vi "Dashboard Main.vi"() -> ()   [LabVIEW 2018]
uses:
  CustomThings/Routine.ctl
  CustomThings/StartingLocation.ctl
  CustomThings/Height.ctl
  CustomThings/Piece.ctl
  CustomThings/NumberOfPiecesToScore.ctl
  <vilib>/Rock Robotics/WPI/Camera/WPI_CameraExposure Values.ctl
  <vilib>/Rock Robotics/WPI/Camera/WPI_CameraWhite Balance Values.ctl
  <vilib>/Utility/miscctls.llb/LVRowAndColumnTypeDef.ctl
  <vilib>/event_ctls.llb/eventvkey.ctl
  <vilib>/Rock Robotics/Network Tables/NT Read Numeric Array.vi
  <vilib>/Rock Robotics/WPI/Dashboard/WPI_DashboardLogging Global.vi
  <vilib>/Rock Robotics/Network Tables/NT Write Boolean.vi
  <vilib>/Rock Robotics/Network Tables/NT Read Boolean.vi
panel:
  out "NT Connection":bool
  in  "Camera Settings Right":T1={"Frame Rate"=15, "Compression"=30, "Size"=1, "DB Camera Config"=FALSE} {"Frame Rate" scale=1.0..30.0; "Compression" scale=100.0..-1.0; "Size" items=["640x480", "320x240", "160x120"]}
  in  "Camera Name Right":string(combo)="No Camera Selection"
  out "Camera Perf":string="                          "
  in  "Camera Settings":T1={"Frame Rate"=10, "Compression"=66, "Size"=2, "DB Camera Config"=FALSE} {"Frame Rate" scale=1.0..30.0; "Compression" scale=100.0..-1.0; "Size" items=["640x480", "320x240", "160x120"]}
  in  "TCP":refnum<k5>
  in  "Rec Mode":enum32{"Stop", "Record", "Playback"}(radio)
  out "Robot IP":string
  out "Image Message":string="Timeout in Camera Communications"
  in  "Dashboard Tab":T2(tab)=enum."Custom"
  out "LEDs":u32(colorbox)
  out "ArmHeight":dbl(slide) scale=0.0..100.0
  out "HatchLimitSwitch":bool
  out "LimitSwitchBottom":bool
  out "LimitSwitchTop":bool
  out "Mode":T3(ring)=enum."Disconnected"
  out "Right Camera Perf":cluster{"Bandwidth (Mbps)":dbl, "FPS":dbl}
  in  "Reset":bool
  out "LeftEncoder":dbl
  out "RightEncoder":dbl
  out "Gyro":dbl(knob) scale=-180.0..180.0
  in  "Pieces  to Score":T4=enum."3"
  in  "Rocket Level":T5
  in  "Delay":dbl
  in  "Starting Position":T6
  in  "Routine":T7
  in  "Battery Number":string
  out "Starting Piece":T8=enum."Hatch Panel"
  out "Camera Image Right":T9(plugin-control)
  in  "DB/String 9":string
  in  "DB/String 8":string
  in  "DB/String 7":string
  in  "DB/String 6":string
  in  "DB/String 5":string
  in  "DB/String 4":string
  in  "DB/String 3":string
  in  "DB/String 2":string
  in  "DB/String 1":string
  in  "DB/String 0":string
  in  "DB/Slider 0":dbl(slide) scale=0.0..5.0
  in  "DB/Slider 1":dbl(slide) scale=0.0..5.0
  in  "DB/Slider 2":dbl(slide) scale=0.0..5.0
  in  "DB/Slider 3":dbl(slide) scale=0.0..5.0
  out "DB/LED 3":bool
  out "DB/LED 2":bool
  out "DB/LED 1":bool
  out "DB/LED 0":bool
  in  "DB/Button 3":bool
  in  "DB/Button 2":bool
  in  "DB/Button 1":bool
  in  "DB/Button 0":bool caption="New Name"
  in  "Test Slider":dbl(slide) scale=0.0..100.0 scale format="%#_3g"
  in  "On/Off":bool caption="Solenoid"
  in  "Test Name":u16(ring) items=["Select the test to run..."]
  in  "Test Tree":string(tree)
  in  "Motor":cluster{"Value":dbl, "Enable":bool} {"Value" scale=-1.0..1.0 scale format="%#_3g"}
  out "Progress":T10 {"Test Progress" scale=0.0..100.0}
  in  "Rev/Fwd":cluster{"Forward":bool, "Reverse":bool}
  in  "Test Ring":u16(ring) items=["Monochrome", "Color"]
  out "Cmd Status":string
  in  "Execute Command":bool
  in  "Command Params":string[][](table)
  in  "Command Selection":i32(listbox)
  in  "CheckList":i32(listbox)
  out "Tree":string(tree)
  out "Camera Image":T9(plugin-control)
  in  "Camera Name":string(combo)="No Camera Selection"
  # "HW"
  # "HW"
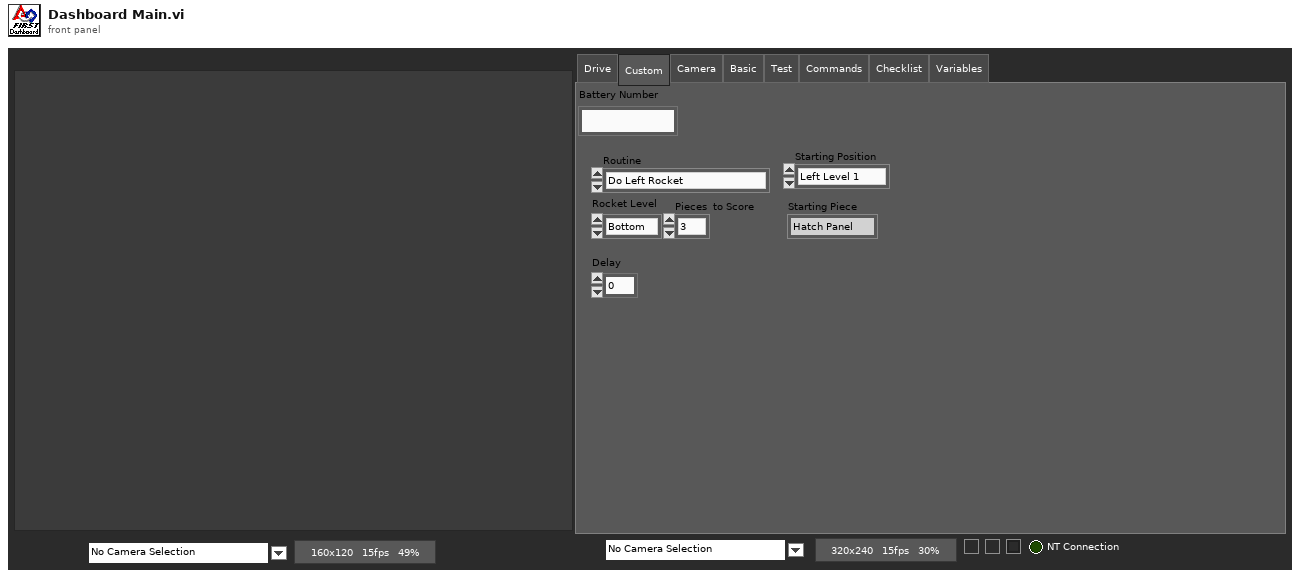
[diagram p1: front panel]
types:
  T1 = cluster{"Frame Rate":i32, "Compression":i32, "Size":u16, "DB Camera Config":bool}
  T2 = enum32{"Drive", "Custom", "Camera", "Basic", "Test", "Commands", "Checklist", "Variables"}
  T3 = enum8{"Tele-Op Disabled", "Tele-Op Enabled", "Auto Disabled", "Auto Enabled", "Test Disabled", "Test Enabled", "Disconnected", "No Code", "E-Stop"}
  T4 = typedef "NumberOfPiecesToScore.ctl" = enum16{"1", "2", "3", "4"}
  T5 = typedef "Height.ctl" = enum16{"Bottom", "Middle", "Top"}
  T6 = typedef "StartingLocation.ctl" = enum16{"Left Level 1", "Center Level 1", "Right Level 1", "Left Level 2", "Right Level 2"}
  T7 = typedef "Routine.ctl" = enum16{"Do Left Rocket", "Do Right Rocket", "Do Left Cargo Ship Panels", "Do Right Cargo Ship Panels", "Do Front Left Cargo Ship", "Do Front Right Cargo Ship", "Do Teleop"}
  T8 = typedef "Piece.ctl" = enum16{"None", "Cargo", "Hatch Panel"}
  T9 = typedef "IMAQ Image.ctl" = refnum<image>
  T10 = cluster{"Test Progress":u8, "Test Progress Text":string}
  T11 = cluster{"Save Path":path, "Interval (s)":dbl, "Keep":i32}
  T12 = typedef "Image Type" = u32
  T13 = cluster{"IDs":cluster{"RPC field ID":u16, "Unique ID":u16}, "String":string}
  T14 = cluster{"Error Strings":string, "Disable Counts":cluster{u16, u16}, "Rail Faults":cluster{u16, u16, u16}, "Robot IP":string, "DB Mode":u8, "Event Info":cluster{"Name":string, "Type":u8, "Number":u16, "Replay":u8}}
  T15 = cluster{"Storage":cluster{"Disk Free":u64, "RAM Block":u32, "RAM free":u32}, "CPU Utilization":cluster{"CPU % ISR":sgl, "CPU % Time Crit":sgl, "CPU % Timed Str":sgl, "CPU % High":sgl, "CPU % Above":sgl, "CPU % Normal":sgl, "CPU % Low":sgl}, "CAN":cluster{"% Bus Utilization":sgl, "Bus Off Cnt":u32, "TX_FIFO Full Cnt":u32, "Receive Error Cnt":u8, "Transmit Error Cnt":u8}, "HID":cluster{"HID Outputs":u32, "Rumble Low":u16, "Rumble High":u16}[]}
  T16 = cluster{"Status bits":cluster{"Test Mode":bool, "Autonomous":bool, "Enabled":bool, "Code Start":bool, "Brownout":bool, "Reserved 2":bool, "Reserved 3":bool, "E-Stop":bool}, "Code Trace":cluster{"Disabled":bool, "TeleOp":bool, "Auto":bool, "Test":bool}, "Controller Type":enum16{"unknown", "cRIO", "roboRio"}, "Code?":enum16{"unknown", "noCode", "code"}, "Battery V":dbl}
  T17 = cluster{"Control Bits":cluster{"TestMode":bool, "Autonomous":bool, "Enabled":bool, "FMS Present":bool, bool, bool, bool, "E-Stop":bool}, "Team Station ":u8, "Countdown":sgl, "Joystick Values":cluster{"Axes":dbl[], "Buttons":bool[], "POVs":i16[]}[]}
  T18 = cluster{"Axes":dbl[], "Buttons":bool[], "POVs":i16[]}[]
  T19 = cluster{"Axes":dbl[], "Buttons":bool[], "POVs":i16[]}
  T20 = cluster{"Camera Image":refnum<vi>, "Dashboard Tab":refnum<vi>, "Rec Mode":refnum<vi>, "Test Slider":refnum<vi>, "On/Off ":refnum<vi>, "Test Ring":refnum<vi>, "Rev/Fwd":refnum<vi>, "Test Name":refnum<vi>, "Motor":refnum<vi>, "Progress":refnum<vi>, "CheckList":refnum<vi>, "Tree":refnum<vi>, "Test Tree":refnum<vi>, "Command Params":refnum<vi>, "Command Selection":refnum<vi>, "Execute Command":refnum<vi>, "Cmd Status":refnum<vi>, "Camera Settings":refnum<vi>, "Camera Name":refnum<vi>, "Camera Perf":refnum<vi>, "Camera Settings Right":refnum<vi>, "Camera Name Right":refnum<vi>, "Camera Image Right":refnum<vi>}
  T21 = typedef "WPI_CameraExposure Values.ctl" = enum16{"Auto", "Flicker-free 50 Hz", "Flicker-free 60 Hz", "Hold current", "Custom"}
  T22 = typedef "WPI_CameraWhite Balance Values.ctl" = enum16{"Auto", "Fixed indoor", "Fixed outdoor 1", "Fixed outdoor 2", "Fixed fluorescent 1", "Fixed fluorescent 2", "Hold current", "Custom"}
  T23 = cluster{"Exposure":T21, "Exposure (%)":dbl, "Brightness":i32, "White Balance":T22, "Color Temp (K)":dbl}
  T24 = cluster{"Global Rectangle":i32[], "Contours":cluster{"Contour Type":u32, "ROI Type":u32, "Points":i32[]}[]}
  T25 = cluster{"Camera Name":string, string, "Saved DB Images Info":cluster{"Save Path":path, "Interval (s)":dbl, "Keep":i32}}
  T26 = cluster{"Camera Name Right":string, string, "Saved DB Images Info":cluster{"Save Path":path, "Interval (s)":dbl, "Keep":i32}}
  T27 = cluster{"Operation":enum16{"Update", "Clear"}, "Color Box":u32}[]
  T28 = typedef "eventvkey.ctl" = enum16{"ASCII", "Enter", "Return", "Shift", "Ctrl", "Alt", "Cmd", "Opt", "Caps", "NumLock", "Clear", "Break", "Up", "Down", "Left", "Right", "Insert", "Delete", "Home", "End", "PageUp", "PageDown", "Escape", "Help", "Pause", "ScrollLock", "F1", "F2", "F3", "F4", "F5", "F6", "F7", "F8", "F9", "F10", "F11", "F12", "F13", "F14", "F15", "F16", "F17", "F18", "F19", "F20", "F21", "F22", "F23", "F24", "Play", "VolumeUp", "VolumeDown", "Mute", "Two Byte Char"}
  T29 = cluster{"Image Size":bool, "Image Type":bool, "Pixel Value":bool, "ROI Information":bool, "Zoom Factor":bool}
  T30 = cluster{"Operation":enum16{"Update", "Clear"}, "Color Box":u32}
  T31 = typedef "LVRowAndColumnTypeDef.ctl" = cluster{"Row":i32, "Column":i32}
  T32 = cluster{"Shift":bool, "Ctrl":bool, "Alt":bool, "Cmd":bool, "Opt":bool}
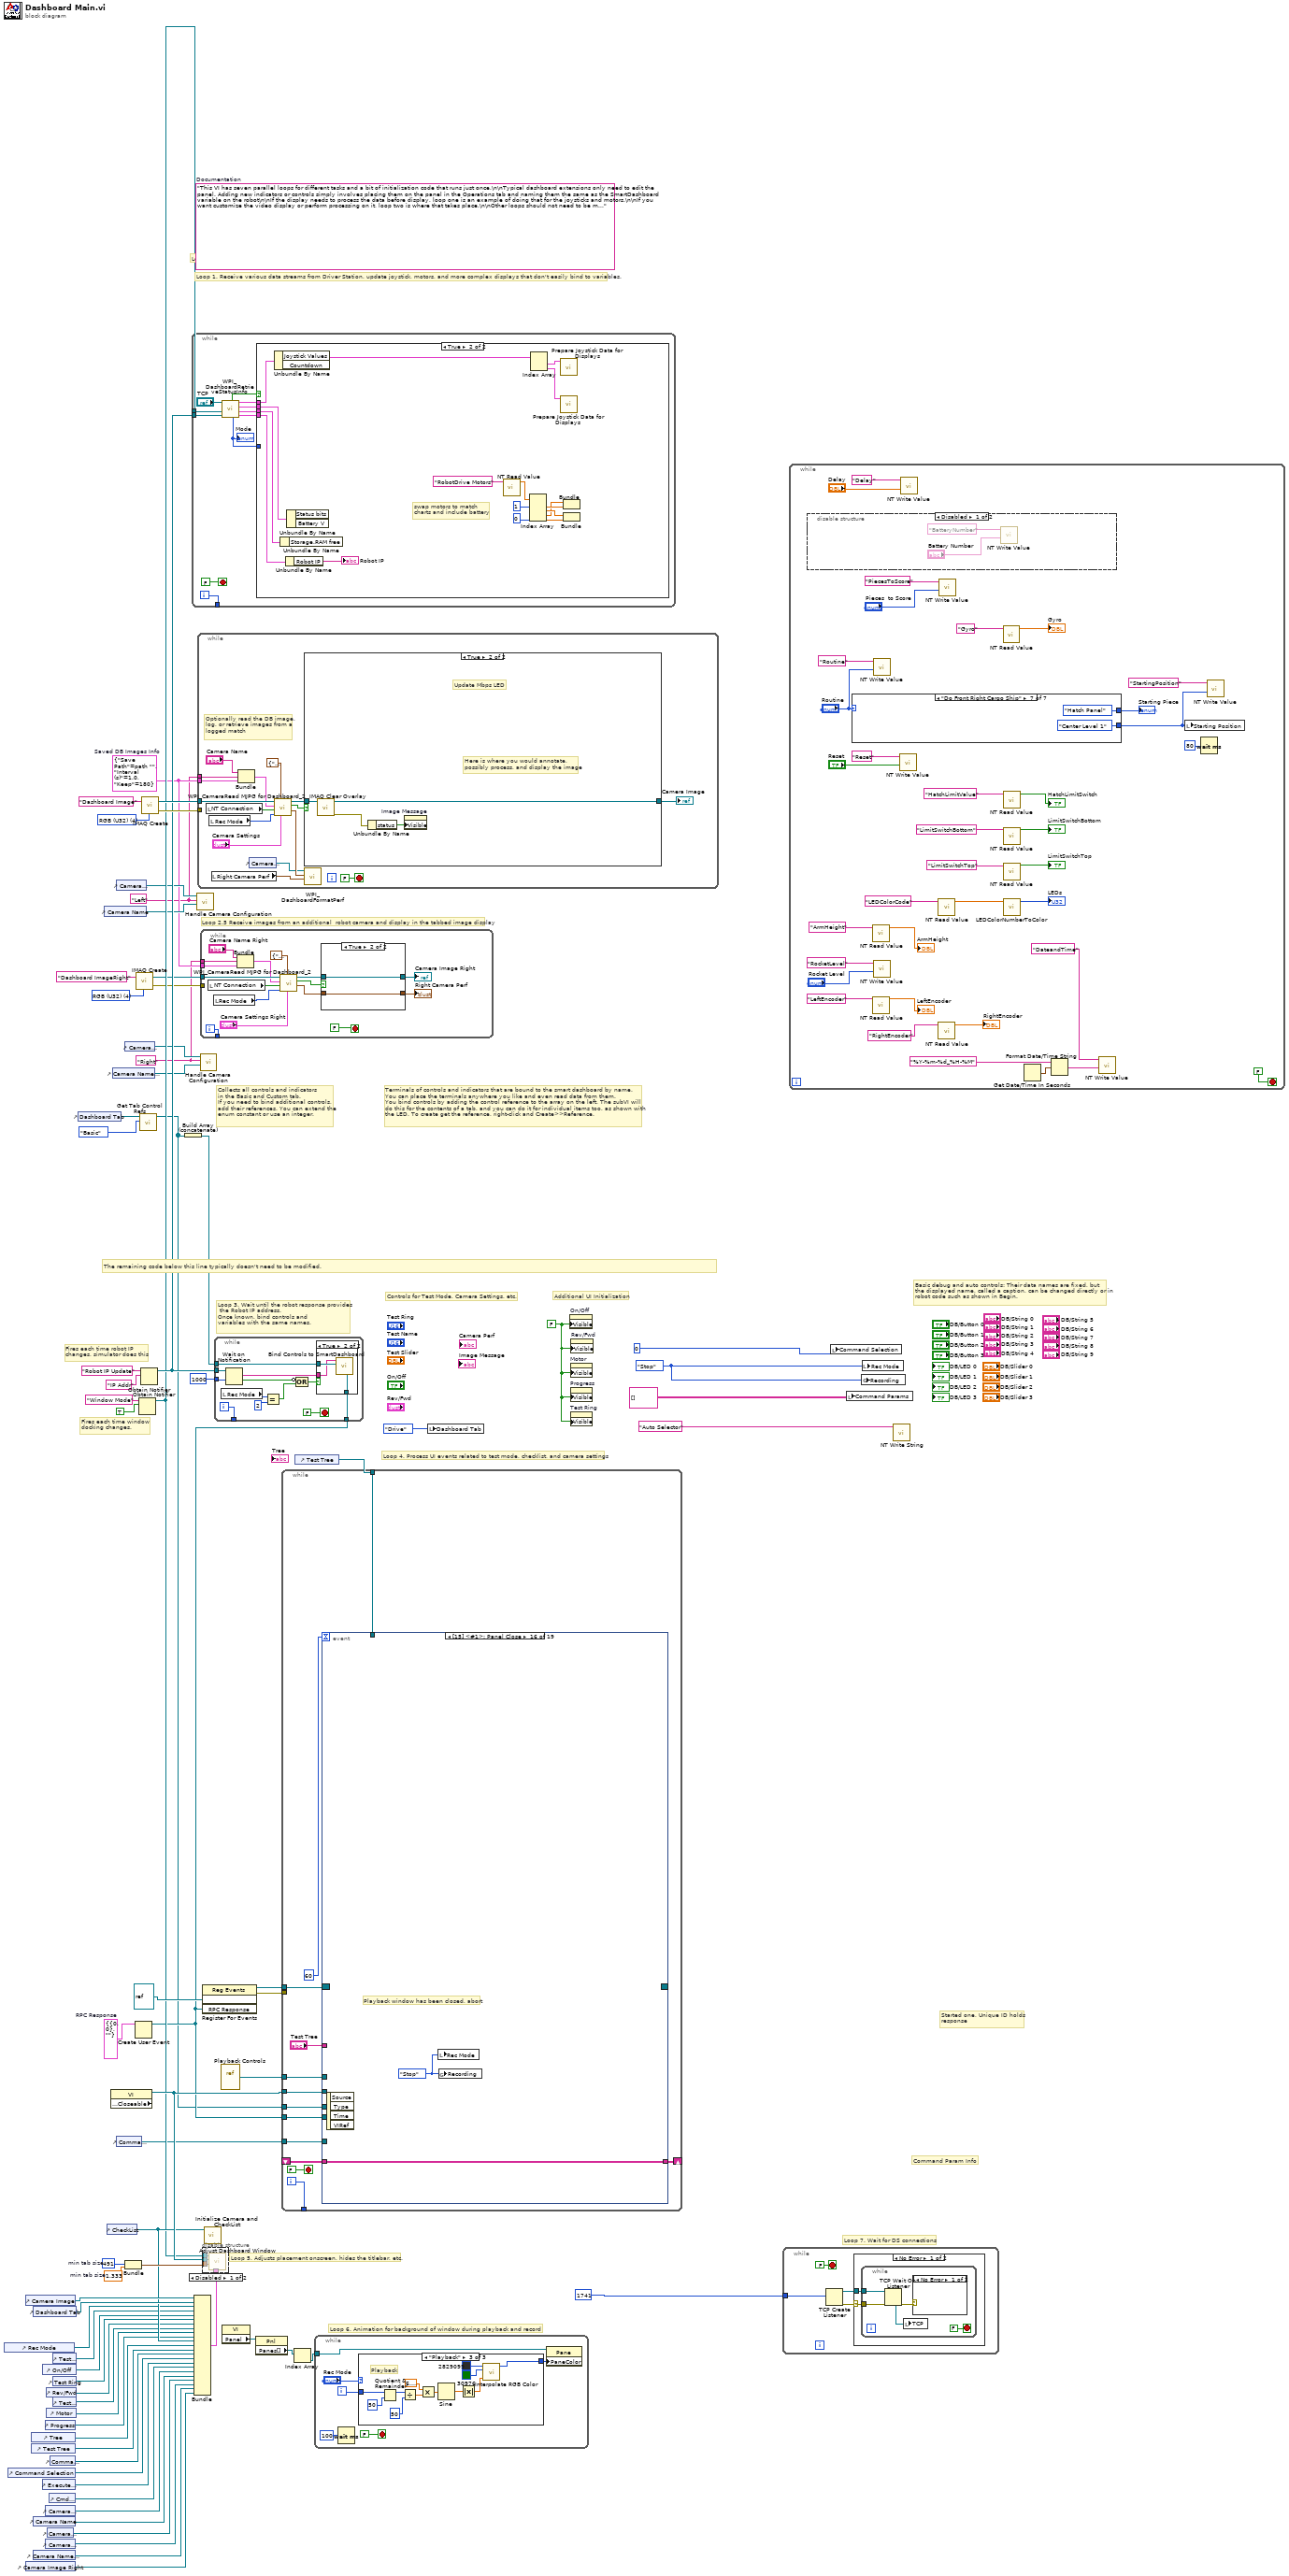
[diagram p0: block diagram]
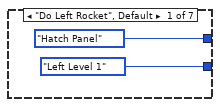
[diagram p2: hidden frame]
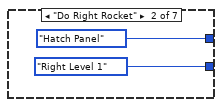
[diagram p3: hidden frame]
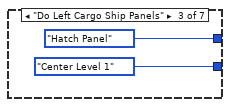
[diagram p4: hidden frame]
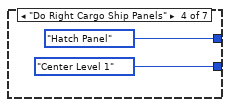
[diagram p5: hidden frame]
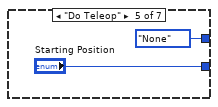
[diagram p6: hidden frame]
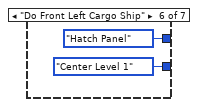
[diagram p7: hidden frame]
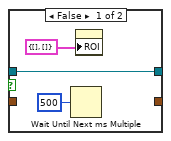
[diagram p10: hidden frame]
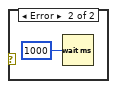
[diagram p11: hidden frame]
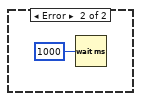
[diagram p12: hidden frame]
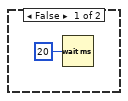
[diagram p13: hidden frame]
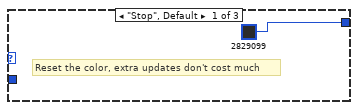
[diagram p14: hidden frame]
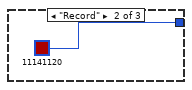
[diagram p15: hidden frame]
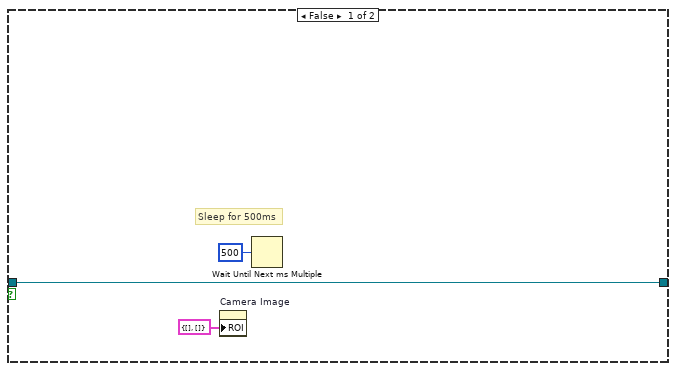
[diagram p17: hidden frame]
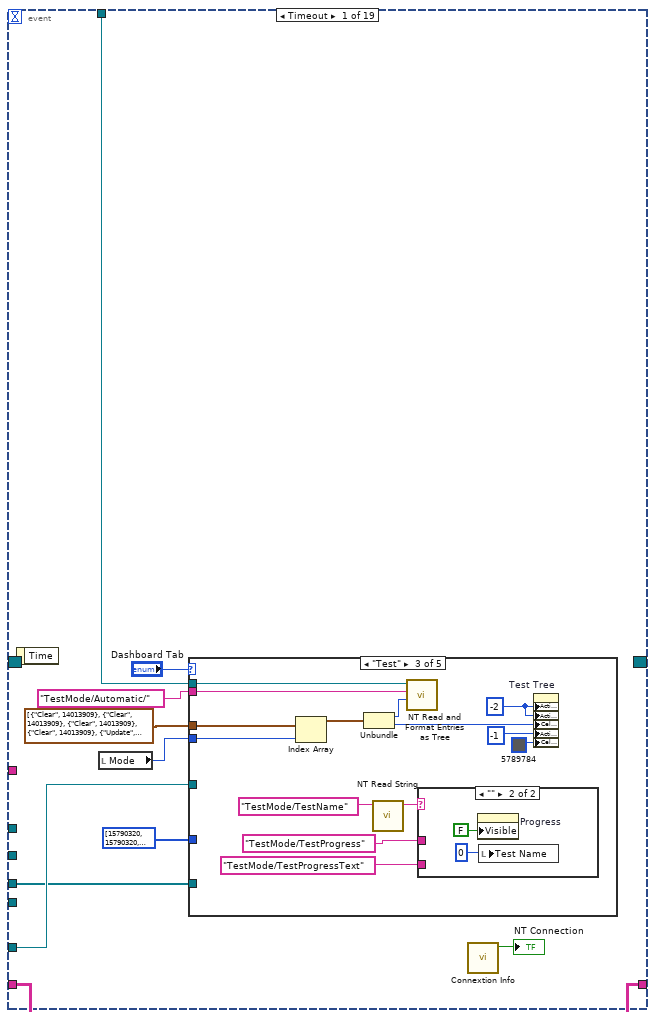
[diagram p18: hidden frame]
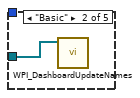
[diagram p20: hidden frame]
diagram:
  w4 = T11 {"Save Path"=path "", "Interval (s)"=1.0, "Keep"=180}  # Saved DB Images Info
  w3 = "Right"
  w2 = "Left"
  w12 = T12 4 items=["Grayscale (U8)", "Grayscale (I16)", "Grayscale (SGL)", "Complex (CSG)", "RGB (U32)", "HSL (U32)", "RGB (U64)"] ("Image Type")
  w27 = T13 {"IDs"={"RPC field ID"=0, "Unique ID"=0}, "String"=""}  # RPC Response
  w49 = 491  # min tab size
  w48 = 1.333  # min tab size
  w55 = enum32{"Stop", "Record", "Playback"}."Stop" ("Rec Mode")
  w34 = FALSE ("Visible")
  (unwired) "This VI has seven parallel loops for different tasks and a bit of initialization code that runs just once.\n\nTypical dashboard extensions only need to edit the panel. Adding new indicators or controls simply involves placing them on the panel in the Operations tab and naming them the same as the SmartDashboard variable on the robot\n\nIf the display needs to process the data before display, loop one is an example of doing that for the joysticks and motors.\n\nIf you want customize the video display or perform processing on it, loop two is where that takes place.\n\nOther loops should not need to be modified. They are pretty standard, and document the task they perform."  # Documentation
  w72 = T12 4 items=["Grayscale (U8)", "Grayscale (I16)", "Grayscale (SGL)", "Complex (CSG)", "RGB (U32)", "HSL (U32)", "RGB (U64)"] ("Image Type")
  # "Loop 2.5 Receive images from an additional  robot camera and display in the tabbed image display"
  # "Command Param Info"
  # "Started one, Unique ID holds\nresponse"
  # "Loop 7. Wait for DS connections"
  # "Basic debug and auto controls: Their data names are fixed, but\nthe displayed name, called a caption, can be changed directly or in\nrobot code such as shown in Begin."
  # "Controls for Test Mode, Camera Settings, etc."
  # "Additional UI Initialization"
  # "Loop 6. Animation for background of window during playback and record"
  # "Fires each time robot IP\nchanges, simulator does this"
  # "Fires each time window\ndocking changes."
  # "Collects all controls and indicators\nin the Basic and Custom tab.\nIf you need to bind additional controls,\nadd their references. You can extend the\nenum constant or use an integer."
  # "The remaining code below this line typically doesn't need to be modified."
  # "Loop 4. Process UI events related to test mode, checklist, and camera settings"
  # "Terminals of controls and indicators that are bound to the smart dashboard by name.\nYou can place the terminals anywhere you like and even read data from them.\nYou bind controls by adding the control reference to the array on the left. The subVI will\ndo this for the contents of a tab, and you can do it for individual items too, as shown with\nthe LED. To create get the reference, right-click and Create>>Reference."
  # "Loop 3. Wait until the robot response provides\n the Robot IP address.\nOnce known, bind controls and\nvariables with the same names."
  # "Loop 5. Adjusts placement onscreen, hides the titlebar, etc."
  # "Loop 1. Receive various data streams from Driver Station, update joystick, motors, and more complex displays that don't easily bind to variables."
  # "Loop 2. Receive primary camera images from robot, update Mbps, fps, and do any processing or display"
  n1 = control-ref of="Rec Mode"() -> (w40:refnum<vi>)
  n2 = control-ref of="Command Selection"() -> (w26:refnum<vi>)
  n3 = control-ref of="Camera Image Right"() -> (w5:refnum<vi>)
  n4 = control-ref of="Camera Image"() -> (w51:refnum<vi>)
  n5 = control-ref of="Tree"() -> (w44:refnum<vi>)
  n6 = control-ref of="Test Tree"() -> (w43:refnum<vi>)
  n7 = control-ref of="Dashboard Tab"() -> (w50:refnum<vi>)
  n8 = control-ref of="Camera Name"() -> (w17:refnum<vi>)
  n9 = control-ref of="Camera Name Right"() -> (w6:refnum<vi>)
  n10 = control-ref of="Execute Command"() -> (w28:refnum<vi>)
  n11 = control-ref of="On/Off"() -> (w38:refnum<vi>)
  n12 = control-ref of="Progress"() -> (w35:refnum<vi>)
  n13 = control-ref of="Camera Settings"() -> (w18:refnum<vi>)
  n14 = control-ref of="Camera Settings Right"() -> (w7:refnum<vi>)
  n15 = control-ref of="Rev/Fwd"() -> (w36:refnum<vi>)
  n16 = control-ref of="Motor"() -> (w41:refnum<vi>)
  n17 = control-ref of="Camera Perf"() -> (w16:refnum<vi>)
  n18 = control-ref of="Cmd Status"() -> (w22:refnum<vi>)
  n19 = control-ref of="Command Params"() -> (w29:refnum<vi>)
  n20 = control-ref of="Test Slider"() -> (w39:refnum<vi>)
  n21 = control-ref of="Test Ring"() -> (w37:refnum<vi>)
  n22 = control-ref of="Test Name"() -> (w42:refnum<vi>)
  n23 = control-ref of="Dashboard Tab"() -> (w53:refnum<vi>)
  n24 = control-ref of="Camera Name"() -> (w19:refnum<vi>)
  n25 = control-ref of="CheckList"() -> (w45:refnum<vi>)
  n26 = property class="VI" props=["Front Panel.Closeable"]() -> (reference out=w54:refnum<vi>)  [unwired: 2 in, 2 out]
  n27 = control-ref of="Camera Name Right"() -> (w8:refnum<vi>)
  n28 = control-ref of="Camera Settings"() -> (w20:refnum<vi>)
  n29 = control-ref of="Command Params"() -> (w21:refnum<vi>)
  n30 = control-ref of="Camera Settings Right"() -> (w9:refnum<vi>)
  n31 = Bundle("min tab size"=w49, "min tab size"=w48) -> (w47:cluster{"min tab size":i32, "min tab size":dbl})  [unwired: 1 in]
  n32 = Create User Event(user event datatype=w27) -> (user event=w23:refnum<user-event>)  [unwired: 1 in, 1 out]
  n33 = call "IMAQ Create"("Image Name"="Dashboard ImageRight", "Image Type"=w12) -> ("New Image"=w11:T9, "error out"=w10:errorcluster)  [unwired: 2 in, 1 out]
  n34 = Obtain Notifier(name (unnamed)="Window Mode", notification data type=TRUE) -> (notifier out=w32:refnum<notifier>)  [unwired: 2 in, 2 out]
  n35 = call <vilib>:"Get Tab Control Refs.vi"("Page Index"=T2."Basic" ("Dashboard Tab"), "TabControl in"=w53) -> ("ControlsOnPage"=w15:refnum<vi>[])  [unwired: 9 in]
  n36 = Obtain Notifier(name (unnamed)="Robot IP Update", notification data type="IP Addr" ("name (unnamed)")) -> (notifier out=w33:refnum<notifier>)  [unwired: 2 in, 2 out]
  n37 = call "IMAQ Create"("Image Name"="Dashboard Image", "Image Type"=w72) -> ("New Image"=w70:T9, "error out"=w69:errorcluster)  [unwired: 2 in, 1 out]
  n38 = Build Array (concatenate)(w15) -> (w52:refnum<vi>[])
  n39 = while {
    tunnel: [w82] -> _
    tunnel: w33 -> [w76]
    tunnel: w32 -> [w73]
    i -> [w82]
    stop <- FALSE stop-if-true
    n40 = call <vilib>:"WPI_DashboardRetrieveStatusInfo.vi"("Binding Refnum"=w76, "Window Mode Notifier"=w73, "TCP Cnx"="TCP") -> ("Power and Errors"=w77:T14, "Robot Metrics"=w80:T15, "Status Info"=w81:T16, "Control Info"=w78:T17, "Robot Mode"=w75:T3, "Process?"=w79:bool)  [unwired: 3 in]
    "Mode" <- w75
    n41 = case shown="True" w79 {
      tunnel: w81 -> [_ w100]
      tunnel: w80 -> [_ w99]
      tunnel: w78 -> [_ w98]
      tunnel: w77 -> [_ w97]
      tunnel: w75 -> [_ _]
      frame False {
        n42 = Wait (ms)(milliseconds to wait=u32 20) -> ()  [unwired: 1 out]
      }
      frame True {
        # "swap motors to match\ncharts and include battery"
        n43 = Unbundle By Name(w98) -> ("Joystick Values"=w90:T18)  [unwired: 1 out]
        n44 = Unbundle By Name(w99) -> ()  [unwired: 1 out]
        n45 = Unbundle By Name(w97) -> ("Robot IP"=→"Robot IP":string)
        n46 = Unbundle By Name(w100) -> ()  [unwired: 2 out]
        n47 = call-poly <vilib>:"NT Read Value.vi"("Name"="RobotDrive Motors") -> ("Numeric Array"=w86:dbl[])  [unwired: 9 in, 1 out]
        n48 = Index Array(array=w86, index #1=1, index #4=0) -> (element #1=w92:dbl, element #2=w93:dbl, element #3=w91:dbl, element #4=w96:dbl)  [unwired: 2 in]
        n49 = Index Array(array=w90) -> (element #1=w89:T19, element #2=w88:T19)  [unwired: 2 in]
        n50 = call "Prepare Joystick Data for Displays.vi"("Joystick Values"=w88) -> ()  [unwired: 8 in, 3 out]
        n51 = call "Prepare Joystick Data for Displays.vi"("Joystick Values"=w89) -> ()  [unwired: 8 in, 3 out]
        n52 = Bundle("Numeric"=w91, "Numeric"=w92) -> ()  [unwired: 1 in, 1 out]
        n53 = Bundle("Numeric"=w93, "Numeric"=w96) -> ()  [unwired: 1 in, 1 out]
      }
    }
  }
  n54 = Bundle("Camera Image"=w51, "Dashboard Tab"=w50, "Rec Mode"=w40, "Test Slider"=w39, "On/Off"=w38, "Test Ring"=w37, "Rev/Fwd"=w36, "Test Name"=w42, "Motor"=w41, "Progress"=w35, "CheckList"=w45, "Tree"=w44, "Test Tree"=w43, "Command Params"=w29, "Command Selection"=w26, "Execute Command"=w28, "Cmd Status"=w22, "Camera Settings"=w18, "Camera Name"=w17, "Camera Perf"=w16, "Camera Settings Right"=w7, "Camera Name Right"=w6, "Camera Image Right"=w5) -> (w46:T20)  [unwired: 1 in]
  n55 = call "Handle Camera Configuration.vi"("CameraNameRef"=w19, "Display Name"=w2, "ClusterRef"=w20) -> ()  [unwired: 9 in]
  n56 = while {
    tunnel: w70 -> [w115]
    tunnel: w69 -> [_]
    tunnel: w4 -> [w108]
    tunnel: w2 -> [w105]
    stop <- FALSE stop-if-true
    # "Optionally read the DB image,\nlog, or retrieve images from a\nlogged match"
    n57 = local read "NT Connection"() -> (w109:bool)
    n58 = local read "Rec Mode"() -> (w112:enum32{"Stop", "Record", "Playback"})
    n59 = local read "Right Camera Perf"() -> (w103:cluster{"Bandwidth (Mbps)":dbl, "FPS":dbl})
    n60 = Bundle("Camera Name"="Camera Name", w105, "Saved DB Images Info"=w108) -> (w107:T25)  [unwired: 1 in]
    n61 = control-ref of="Camera Perf"() -> (w102:refnum<vi>)
    n62 = call <vilib>:"WPI_CameraRead MJPG for Dashboard_2.vi"("Camera Settings"="Camera Settings", "Camera Settings 2"=T23 {"Exposure"=enum."Custom", "Exposure (%)"=75.0, "Brightness"=50, "White Balance"=enum."Custom", "Color Temp (K)"=0.0}, "Rec Mode"=w112, "NT Connection"=w109, "Capture Info"=w107, "Image in"=w115) -> ("perf info"=w104:cluster{"Bandwidth (Mbps)":dbl, "fps":dbl}, "Active"=w113:bool, "Image\\ out"=w114:T9)  [unwired: 3 in]
    n63 = case shown="True" w113 {
      tunnel: w114 -> [w118 w121]
      tunnel: [w118 w120] -> w110
      frame False {
        # "Sleep for 500ms"
        n64 = property on="Camera Image" class="ImageControl"("ROI"=T24 {"Global Rectangle"=[], "Contours"=[]}) -> ()  [unwired: 2 in, 2 out]
        n65 = Wait Until Next ms Multiple(millisecond multiple=u32 500) -> ()  [unwired: 1 out]
      }
      frame True {
        # "Here is where you would annotate,\npossibly process, and display the image"
        # "Update Mbps LED"
        n66 = call "IMAQ Clear Overlay"("Image"=w121) -> ("error out"=w122:errorcluster, "Image Out"=w120:T9)  [unwired: 2 in, 7 out]
        n67 = Unbundle By Name(w122) -> ("status"=w123:bool)
        n68 = property on="Image Message" class="Str"("Visible"=w123) -> ()  [unwired: 2 in, 2 out]
      }
    }
    "Camera Image" <- w110
    n69 = call <vilib>:"WPI_DashboardFormatPerf.vi"("Right Camera Perf"=w103, "Performance"=w104, "String in"=w102) -> ()  [unwired: 9 in]
  }
  n70 = while {
    tunnel: w11 -> [w139]
    tunnel: w10 -> [_]
    tunnel: [w134] -> _
    tunnel: w4 -> [w130]
    tunnel: w3 -> [w127]
    i -> [w134]
    stop <- FALSE stop-if-true
    n71 = local read "NT Connection"() -> (w131:bool)
    n72 = local read "Rec Mode"() -> (w138:enum32{"Stop", "Record", "Playback"})
    n73 = Bundle("Camera Name Right"="Camera Name Right", w127, "Saved DB Images Info"=w130) -> (w129:T26)  [unwired: 1 in]
    n74 = call <vilib>:"WPI_CameraRead MJPG for Dashboard_2.vi"("Camera Settings"="Camera Settings Right", "Camera Settings 2"=T23 {"Exposure"=enum."Custom", "Exposure (%)"=75.0, "Brightness"=50, "White Balance"=enum."Custom", "Color Temp (K)"=0.0}, "Rec Mode"=w138, "NT Connection"=w131, "Capture Info"=w129, "Image in"=w139) -> ("perf info"=w125:cluster{"Bandwidth (Mbps)":dbl, "fps":dbl}, "Active"=w133:bool, "Image\\ out"=w136:T9)  [unwired: 3 in]
    n75 = case shown="True" w133 {
      tunnel: w136 -> [w141 w144]
      tunnel: [w141 w144] -> w132
      tunnel: [_ w143] -> w126
      tunnel: w125 -> [_ w143]
      frame False {
        n76 = Wait Until Next ms Multiple(millisecond multiple=u32 500) -> ()  [unwired: 1 out]
        n77 = property on="Camera Image Right" class="ImageControl"("ROI"=T24 {"Global Rectangle"=[], "Contours"=[]}) -> ()  [unwired: 2 in, 2 out]
      }
      frame True {
      }
    }
    "Camera Image Right" <- w132
    "Right Camera Perf" <- w126
  }
  n78 = call "Handle Camera Configuration.vi"("CameraNameRef"=w8, "Display Name"=w3, "ClusterRef"=w9) -> ()  [unwired: 9 in]
  n79 = register-events(refnum<vi> refnum, w23) -> (reference out=w59:refnum<event-registration>, error out=w58:errorcluster)  [unwired: 2 in]
  n80 = disable-structure shown="Disabled" {
    disable-tunnel: w54 -> [w148 _]
    disable-tunnel: w47 -> [w147 _]
    disable-tunnel: w46 -> [w146 _]
    disable-tunnel: w32 -> [w145 _]
    frame Disabled {
      n81 = call "Adjust Dashboard Window.vi"("Sizing Refnums"=w146, "Size Constraints"=w147, "VI"=w148, "WIn Mode"=w145) -> ()  [unwired: 8 in]
    }
    frame Enabled {
    }
  }
  n82 = call "Initialize Camera and CheckList.vi"("ListBox in"=w45) -> ()  [unwired: 11 in]
  n83 = while {
    tunnel: w52 -> [w160]
    tunnel: w33 -> [w158]
    tunnel: [w156] -> _
    tunnel: u32 1000 ("milliseconds to wait") -> [w155]
    tunnel: w23 -> [w149]
    i -> [w156]
    stop <- FALSE stop-if-true
    n84 = local read "Rec Mode"() -> (w151:enum32{"Stop", "Record", "Playback"})
    n85 = Wait on Notification(notifier=w158, timeout in ms (-1)=w155) -> (notification=w157:string, timed out?=w153:bool)  [unwired: 2 in, 2 out]
    n86 = Equal?(x=w151, y=u16 2 ("Rec Mode")) -> (x = y?=w152:bool)
    n87 = Compound Arithmetic op=OR(invert w153, w152) -> (w154:bool)
    n88 = case shown="True" w154 {
      tunnel: w160 -> [_ w163]
      tunnel: w157 -> [_ w162]
      tunnel: w149 -> [_ w161]
      frame False {
      }
      frame True {
        n89 = call <vilib>:"Bind Controls to SmartDashboard.vi"("RPC ref"=w161, "Bound Control Refs"=w163, "Server IP Address"=w162) -> ()  [unwired: 9 in]
      }
    }
  }
  n90 = vi-ref "Playback Controls.vi"() -> (w60:refnum<vi>)
  n91 = property class="VI"() -> ("Panel"=w62:refnum<vi>)  [unwired: 2 in, 2 out]
  n92 = property class="Pnl"(reference=w62) -> ("Panes[]"=w63:refnum<vi>[])  [unwired: 1 in, 2 out]
  n93 = Index Array(array=w63) -> (element=w61:refnum<vi>)  [unwired: 1 in]
  n94 = control-ref of="Test Tree"() -> (w64:refnum<vi>)
  n95 = while {
    tunnel: [w173] -> _
    tunnel: w64 -> [w172]
    tunnel: w60 -> [w171]
    tunnel: w59 -> [w170]
    tunnel: w58 -> [_]
    tunnel: w54 -> [w169]
    tunnel: w23 -> [w168]
    tunnel: w21 -> [w167]
    shift-right: [w166] -> _
    shift-left: _ -> [w165]
    tunnel: w15 -> [w164]
    i -> [w173]
    stop <- FALSE stop-if-true
    n96 = event shown="[15] <#1>: Panel Close" {
      selector: w170 -> [_ _ _ _ _ _ _ _ _ _ _ _ _ _ _ _ _ _ _]
      dyn-events: [_ _ _ _ _ _ _ _ _ _ _ _ _ _ w427 _ _ _ _] -> _
      timeout: u32 60 ("milliseconds to wait") -> [_ _ _ _ _ _ _ _ _ _ _ _ _ _ _ _ _ _ _]
      tunnel: w172 -> [w185 _ _ _ _ _ _ _ _ _ _ _ _ _ _ _ _ _ _]
      tunnel: "Test Tree" -> [_ _ _ _ _ _ _ _ _ w394 w402 w404 w408 w416 _ _ _ _ _]
      tunnel: w171 -> [_ _ _ _ _ _ _ _ _ _ _ _ _ _ w429 _ w447 _ _]
      tunnel: w169 -> [_ _ _ _ _ _ _ _ _ _ _ _ _ _ w425 _ _ _ _]
      tunnel: w168 -> [_ _ _ _ _ _ _ _ _ _ _ _ _ _ w423 _ _ _ _]
      tunnel: w167 -> [w180 _ _ _ w345 _ _ _ _ _ _ _ _ _ _ _ _ _ _]
      tunnel: [w179 w228 w330 w335 w343 w352 w362 w369 w381 w393 w400 w403 w407 w415 w422 w442 w444 w448 w461] -> w166
      tunnel: w165 -> [w179 w228 w330 w335 w343 _ _ w369 w381 w393 w400 w403 w407 w415 w422 w442 w444 w448 w461]
      tunnel: w164 -> [w177 _ _ _ _ _ _ _ _ _ _ _ _ _ _ _ _ _ _]
      event Timeout {
        n97 = event-data() -> ()  [unwired: 1 in, 1 out]
        n98 = local read "Mode"() -> (w182:T3)
        n99 = case shown="\"Test\"" "Dashboard Tab" {
          tunnel: w185 -> [_ _ w201 _ _]
          tunnel: "TestMode/Automatic/" ("Name Pattern") -> [_ _ w200 _ _]
          tunnel: T27 [{"Operation"=enum."Clear", "Color Box"=14013909}, {"Operation"=enum."Clear", "Color Box"=14013909}, {"Operation"=enum."Clear", "Color Box"=14013909}, {"Operation"=enum."Clear", "Color Box"=14013909}, {"Operation"=enum."Update", "Color Box"=14013909}, {"Operation"=enum."Update", "Color Box"=16777215}, {"Operation"=enum."Clear", "Color Box"=14013909}, {"Operation"=enum."Clear", "Color Box"=14013909}, {"Operation"=enum."Clear", "Color Box"=14013909}] -> [_ _ w193 _ w221]
          tunnel: w182 -> [_ _ w192 _ w220]
          tunnel: u32[] [15790320, 15790320, 15790320, 15790320, 16777215, 16777215, 15790320, 15790320, 15790320] -> [_ _ _ _ w226]
          tunnel: w180 -> [_ _ _ _ w214]
          tunnel: w177 -> [_ w187 _ _ _]
          frame "Custom", Default {
          }
          frame "Basic" {
            n100 = call <vilib>:"WPI_DashboardUpdateNames.vi"("Controls on Tab"=w187) -> ()  [unwired: 11 in]
          }
          frame "Test" {
            w199 = -2 ("Active Item:Row Number")
            n101 = Index Array(array=w193, index=w192) -> (element=w194:T30)
            n102 = Unbundle(w194) -> ("Operation"=w195:enum16{"Update", "Clear"}, "Color Box"=w196:u32)
            n103 = call <vilib>:"NT Read String.vi"("Name"="TestMode/TestName") -> ("String"=w190:string)  [unwired: 9 in, 1 out]
            n104 = call <vilib>:"NT Read and Format Entries as Tree.vi"("Operation"=w195, "Name Pattern"=w200, "Tree Refnum"=w201) -> ()  [unwired: 7 in, 2 out]
            n105 = case shown="\"\"" w190 {
              tunnel: "TestMode/TestProgress" ("Name") -> [w203 _]
              tunnel: "TestMode/TestProgressText" ("Name") -> [w202 _]
              frame Default {
                n106 = call <vilib>:"NT Read Number.vi"("Name"=w203) -> ("Numeric"=w204:dbl)  [unwired: 9 in, 1 out]
                n107 = call <vilib>:"NT Read String.vi"("Name"=w202) -> ("String"=w205:string)  [unwired: 9 in, 1 out]
                n108 = Bundle("Numeric"=w204, "String"=w205) -> (→"Progress":cluster{"Numeric":dbl, "String":string})  [unwired: 1 in]
              }
              frame "" {
                n109 = property on="Progress" class="Clust (strict)"("Visible"=FALSE) -> ()  [unwired: 2 in, 2 out]
                n110 = local write "Test Name"(u16 0) -> ()
              }
            }
            n111 = property on="Test Tree" class="Tree (strict)"("Active Item Row Number"=w199, "ActiveColNum"=w199, "CellBG"=w196, "Active Item Row Number"=-1 ("Active Item:Row Number"), "CellBG"=u32 5789784 ("Color Box")) -> ()  [unwired: 2 in, 2 out]
          }
          frame "Variables" {
            w211 = string[] ["CameraPublisher", "Usage", "DB"]  # Items to initially close
            n112 = First Call?() -> (First Call?: T/F=w212:bool)
            n113 = control-ref of="Tree"() -> (w213:refnum<vi>)
            n114 = Select(t=w211, s=w212, f=string[] []) -> (s? t:f=w209:string[])
            n115 = call <vilib>:"NT Read and Format Entries as Tree.vi"("Tags to  Close"=w209, "Tree Refnum"=w213) -> ()  [unwired: 8 in, 2 out]
          }
          frame "Commands" {
            w222 = u32 5789784 ("Color Box")
            w223 = T31 {"Row"=-1, "Column"=-2} ("Active Cell:Active Cell")
            w225 = T31 {"Row"=-2, "Column"=-2} ("Active Cell:Active Cell")
            n116 = Index Array(array=w226, index=w220) -> (element=w224:u32)
            n117 = Index Array(array=w221, index=w220) -> (element=w219:T30)
            n118 = Unbundle(w219) -> ("Operation"=w218:enum16{"Update", "Clear"})  [unwired: 1 out]
            n119 = local read "Command Selection"() -> (w217:i32)
            n120 = property on="Command Selection" class="MCListbox (strict)"("ActiveCell"=w225, "CellBG"=w224, "ActiveCell"=w223, "CellBG"=w222) -> ()  [unwired: 2 in, 2 out]
            n121 = call <vilib>:"WPI_DashboardUpdate RPC Info.vi"("Operation"=w218) -> ("update"=w216:bool, "commands"=w215:string[][])  [unwired: 9 in]
            n122 = property on="Command Selection" class="MCListbox (strict)"("ItemNames"=w215) -> ()  [unwired: 2 in, 2 out]
            n123 = property on="Command Params" class="Tbl (strict)"("Active Cell"=w225, "Cell BG Color"=w224, "Active Cell"=w223, "Cell BG Color"=w222) -> ()  [unwired: 2 in, 2 out]
            n124 = call <vilib>:"WPI_DashboardUpdate Command Params.vi"("Update"=w216, "NewVal"=w217, "Commands"=w215, "Param Tbl"=w214) -> ()  [unwired: 7 in, 1 out]
          }
        }
        n125 = call <vilib>:"Connextion Info.vi"() -> ("Connected"=→"NT Connection":bool)  [unwired: 10 in, 1 out]
      }
      event "Test Tree": Value Change {
        # "Show appropriate\ncontrols"
        n126 = event-data() -> ("CtlRef"=w231:refnum<vi>, "NewVal"=w229:string)  [unwired: 1 in]
        n127 = call <vilib>:"WPI_UtilitiesGetTreeIOName.vi"("NewVal"=w229, "TreeControl in"=w231) -> ("I/O Name"=w232:string)  [unwired: 9 in]
        n128 = case shown="\"Camera\"" w232 {
          selector: w232 -> [_ w239 _ w261 w270 _]
          tunnel: w229 -> [_ _ w258 w260 _ w277]
          tunnel: cluster{string[]}[] [{["640x480", "320x240", "160x120"]}, {["Auto", "Fixed indoor", "Fixed outdoor 1", "Fixed outdoor 2", "Fixed fluorescent 1", "Fixed fluorescent 2", "Hold current"]}, {["Auto", "Flicker-free 50 Hz", "Flicker-free 60 Hz", "Hold current"]}, {["None", "Prioritize frame rate", "Prioritize image quality"]}, {["Monochrome", "Color"]}] -> [_ _ _ _ _ w276]
          frame Default {
            w234 = FALSE ("Visible")
            w233 = FALSE ("Visible")
            n129 = property on="Motor" class="Clust (strict)"("Visible"=w233) -> ()  [unwired: 2 in, 2 out]
            n130 = property on="Test Ring" class="Ring (strict)"("Visible"=w233) -> ()  [unwired: 2 in, 2 out]
            n131 = property on="Rev/Fwd" class="Clust (strict)"("Visible"=w234) -> ()  [unwired: 2 in, 2 out]
            n132 = property on="On/Off" class="Bool (strict)"("Visible"=w234) -> ()  [unwired: 2 in, 2 out]
            n133 = property on="Test Slider" class="Slide (strict)"("Visible"=w234) -> ()  [unwired: 2 in, 2 out]
          }
          frame "Analog Out", "Motor", "PWM" {
            w240 = FALSE ("Visible")
            n134 = case shown="\"Analog Out\"" w239 {
              tunnel: [1.0 ("Value") -1.0 ("Value") 0.0 ("Value")] -> w238
              tunnel: [255.0 ("Value") 1.0 ("Value") 5.0 ("Value")] -> w237
              tunnel: [128.0 ("Value") 0.0 ("Value") 0.0 ("Value")] -> w236
              tunnel: [64.0 ("Value") 0.5 ("Value") 1.0 ("Value")] -> w235
              frame "PWM" {
              }
              frame "Motor", Default {
              }
              frame "Analog Out" {
              }
            }
            n135 = property on="Motor" class="Clust (strict)"("Visible"=TRUE) -> ()  [unwired: 2 in, 2 out]
            n136 = property on="Value" class="Slide (strict)"("Value"=w236, "Scale.Minimum"=w238, "Scale.Maximum"=w237, "Scale.Increment"=w235) -> ()  [unwired: 2 in, 2 out]
            n137 = property on="On/Off" class="Bool (strict)"("Visible"=w240) -> ()  [unwired: 2 in, 2 out]
            n138 = property on="Test Slider" class="Slide (strict)"("Visible"=w240) -> ()  [unwired: 2 in, 2 out]
            n139 = property on="Test Ring" class="Ring (strict)"("Visible"=w240) -> ()  [unwired: 2 in, 2 out]
            n140 = property on="Rev/Fwd" class="Clust (strict)"("Visible"=w240) -> ()  [unwired: 2 in, 2 out]
          }
          frame "Servo" {
            w256 = FALSE ("Visible")
            n141 = call <vilib>:"NT Read Number.vi"("Name"=w258) -> ("Numeric"=w257:dbl)  [unwired: 9 in, 1 out]
            n142 = property on="Test Slider" class="Slide (strict)"("Visible"=TRUE, "Scale.Maximum"=170.0 ("Scale.Range:Maximum")) -> ()  [unwired: 2 in, 2 out]
            n143 = local write "Test Slider"(w257) -> ()
            n144 = property on="Motor" class="Clust (strict)"("Visible"=w256) -> ()  [unwired: 2 in, 2 out]
            n145 = property on="Rev/Fwd" class="Clust (strict)"("Visible"=w256) -> ()  [unwired: 2 in, 2 out]
            n146 = property on="On/Off" class="Bool (strict)"("Visible"=w256) -> ()  [unwired: 2 in, 2 out]
            n147 = property on="Test Ring" class="Ring (strict)"("Visible"=w256) -> ()  [unwired: 2 in, 2 out]
          }
          frame "Relay", "Solenoid" {
            w259 = FALSE ("Visible")
            n148 = property on="Motor" class="Clust (strict)"("Visible"=w259) -> ()  [unwired: 2 in, 2 out]
            n149 = property on="Test Slider" class="Slide (strict)"("Visible"=w259) -> ()  [unwired: 2 in, 2 out]
            n150 = Search and Replace String(input string=w260, search string="/Value  **", replace string="/Direction") -> (result string=w266:string)  [unwired: 5 in, 3 out]
            n151 = property on="Test Ring" class="Ring (strict)"("Visible"=w259) -> ()  [unwired: 2 in, 2 out]
            n152 = call <vilib>:"NT Read String.vi"("Name"=w266) -> ("String"=w264:string)  [unwired: 9 in, 1 out]
            n153 = Equal?(x="Both directions", y=w264) -> (x = y?=w262:bool)
            n154 = Not(x=w262) -> (.not. x?=w263:bool)
            n155 = property on="Rev/Fwd" class="Clust (strict)"("Visible"=w262) -> ()  [unwired: 2 in, 2 out]
            n156 = property on="On/Off" class="Bool (strict)"("Visible"=w263, "Caption.Text"=w261) -> ()  [unwired: 2 in, 2 out]
          }
          frame "Compressor", "Digital Out" {
            w269 = FALSE ("Visible")
            # "Get direction and finish"
            n157 = property on="Motor" class="Clust (strict)"("Visible"=w269) -> ()  [unwired: 2 in, 2 out]
            n158 = property on="Test Slider" class="Slide (strict)"("Visible"=w269) -> ()  [unwired: 2 in, 2 out]
            n159 = property on="Test Ring" class="Ring (strict)"("Visible"=w269) -> ()  [unwired: 2 in, 2 out]
            n160 = property on="On/Off" class="Bool (strict)"("Visible"=TRUE, "Caption.Text"=w270) -> ()  [unwired: 2 in, 2 out]
            n161 = property on="Rev/Fwd" class="Clust (strict)"("Visible"=FALSE) -> ()  [unwired: 2 in, 2 out]
          }
          frame "Camera" {
            n162 = call <vilib>:"Get Last Path Segment.vi"("String in"=w277) -> ("String out"=w278:string)  [unwired: 10 in]
            n163 = property on="On/Off" class="Bool (strict)"("Visible"=FALSE) -> ()  [unwired: 2 in, 2 out]
            n164 = property on="Motor" class="Clust (strict)"("Visible"=FALSE) -> ()  [unwired: 2 in, 2 out]
            n165 = property on="Rev/Fwd" class="Clust (strict)"("Visible"=FALSE) -> ()  [unwired: 2 in, 2 out]
            n166 = case shown="\"White Balance  **\"" w278 {
              tunnel: w277 -> [w284 w293 w302 w311 w320 _ w326]
              tunnel: w276 -> [w282 w290 w299 w308 w317 _ _]
              frame "Size  **" {
                n167 = Index Array(array=w282) -> (element=w281:cluster{string[]})  [unwired: 1 in]
                n168 = call <vilib>:"NT Read String.vi"("Name"=w284) -> ("String"=w283:string)  [unwired: 9 in, 1 out]
                n169 = Unbundle(w281) -> (w279:string[])
                n170 = Match First String(2:w279, 3:w283) -> (0:w280:i32)  [unwired: 1 out]
                n171 = property on="Test Ring" class="Ring (strict)"("Value"=w280, "Strings []"=w279) -> ()  [unwired: 2 in, 2 out]
                n172 = property on="Test Ring" class="Ring (strict)"("Visible"=TRUE) -> ()  [unwired: 2 in, 2 out]
                n173 = property on="Test Slider" class="Slide (strict)"("Visible"=FALSE) -> ()  [unwired: 2 in, 2 out]
              }
              frame "White Balance  **" {
                n174 = Index Array(array=w290, index=1) -> (element=w291:cluster{string[]})
                n175 = call <vilib>:"NT Read String.vi"("Name"=w293) -> ("String"=w292:string)  [unwired: 9 in, 1 out]
                n176 = Unbundle(w291) -> (w288:string[])
                n177 = Match First String(2:w288, 3:w292) -> (0:w287:i32)  [unwired: 1 out]
                n178 = property on="Test Ring" class="Ring (strict)"("Value"=w287, "Strings []"=w288) -> ()  [unwired: 2 in, 2 out]
                n179 = property on="Test Ring" class="Ring (strict)"("Visible"=TRUE) -> ()  [unwired: 2 in, 2 out]
                n180 = property on="Test Slider" class="Slide (strict)"("Visible"=FALSE) -> ()  [unwired: 2 in, 2 out]
              }
              frame "Exposure  **" {
                n181 = Index Array(array=w299, index=2) -> (element=w300:cluster{string[]})
                n182 = call <vilib>:"NT Read String.vi"("Name"=w302) -> ("String"=w301:string)  [unwired: 9 in, 1 out]
                n183 = Unbundle(w300) -> (w296:string[])
                n184 = Match First String(2:w296, 3:w301) -> (0:w297:i32)  [unwired: 1 out]
                n185 = property on="Test Ring" class="Ring (strict)"("Value"=w297, "Strings []"=w296) -> ()  [unwired: 2 in, 2 out]
                n186 = property on="Test Ring" class="Ring (strict)"("Visible"=TRUE) -> ()  [unwired: 2 in, 2 out]
                n187 = property on="Test Slider" class="Slide (strict)"("Visible"=FALSE) -> ()  [unwired: 2 in, 2 out]
              }
              frame "Exposure Priority  **" {
                n188 = Index Array(array=w308, index=3) -> (element=w309:cluster{string[]})
                n189 = call <vilib>:"NT Read String.vi"("Name"=w311) -> ("String"=w310:string)  [unwired: 9 in, 1 out]
                n190 = Unbundle(w309) -> (w305:string[])
                n191 = Match First String(2:w305, 3:w310) -> (0:w306:i32)  [unwired: 1 out]
                n192 = property on="Test Ring" class="Ring (strict)"("Value"=w306, "Strings []"=w305) -> ()  [unwired: 2 in, 2 out]
                n193 = property on="Test Ring" class="Ring (strict)"("Visible"=TRUE) -> ()  [unwired: 2 in, 2 out]
                n194 = property on="Test Slider" class="Slide (strict)"("Visible"=FALSE) -> ()  [unwired: 2 in, 2 out]
              }
              frame "Color Enable  **" {
                n195 = Index Array(array=w317, index=4) -> (element=w318:cluster{string[]})
                n196 = call <vilib>:"NT Read String.vi"("Name"=w320) -> ("String"=w319:string)  [unwired: 9 in, 1 out]
                n197 = Unbundle(w318) -> (w314:string[])
                n198 = Match First String(2:w314, 3:w319) -> (0:w315:i32)  [unwired: 1 out]
                n199 = property on="Test Ring" class="Ring (strict)"("Value"=w315, "Strings []"=w314) -> ()  [unwired: 2 in, 2 out]
                n200 = property on="Test Ring" class="Ring (strict)"("Visible"=TRUE) -> ()  [unwired: 2 in, 2 out]
                n201 = property on="Test Slider" class="Slide (strict)"("Visible"=FALSE) -> ()  [unwired: 2 in, 2 out]
              }
              frame Default {
                n202 = property on="Test Ring" class="Ring (strict)"("Visible"=FALSE) -> ()  [unwired: 2 in, 2 out]
                n203 = property on="Test Slider" class="Slide (strict)"("Visible"=FALSE) -> ()  [unwired: 2 in, 2 out]
              }
              frame "Brightness  **", "Color Level  **", "Compression  **", "FPS  **", "Sharpness  **" {
                n204 = call <vilib>:"NT Read Number.vi"("Name"=w326) -> ("Numeric"=w325:dbl)  [unwired: 9 in, 1 out]
                n205 = local write "Test Slider"(w325) -> ()
                n206 = property on="Test Slider" class="Slide (strict)"("Visible"=TRUE, "Scale.Maximum"=100.0 ("Scale.Range:Maximum")) -> ()  [unwired: 2 in, 2 out]
                n207 = property on="Test Ring" class="Ring (strict)"("Visible"=FALSE) -> ()  [unwired: 2 in, 2 out]
              }
            }
          }
        }
        n208 = property on="Progress" class="Clust (strict)"("Visible"=FALSE) -> ()  [unwired: 2 in, 2 out]
      }
      event "Test Name": Mouse Enter {
        # "Populate the ring with the list of tests"
        n209 = event-data() -> ()  [unwired: 1 in, 1 out]
        n210 = call <vilib>:"NT Read String Array.vi"("Name"="TestMode/TestList") -> ("String Array"=w334:string[])  [unwired: 9 in, 1 out]
        n211 = Build Array (concatenate)("Select the test to run...", w334) -> (w333:string[])
        n212 = property on="Test Name" class="Ring (strict)"("Strings []"=w333) -> ()  [unwired: 2 in, 2 out]
      }
      event "Test Name": Value Change {
        w336 = FALSE ("Visible")
        # "Tell the robot the test name to run"
        n213 = event-data() -> ("NewVal"=w340:u16)  [unwired: 1 in]
        n214 = property on="Test Name" class="Ring (strict)"() -> ("Strings []"=w341:string[])  [unwired: 2 in, 2 out]
        n215 = local write "Progress"(T10 {"Test Progress"=0, "Test Progress Text"=""} ("Progress")) -> ()
        n216 = Index Array(array=w341, index=w340) -> (element=w339:string)
        n217 = call <vilib>:"NT Write String.vi"("String"=w339, "Name"="TestMode/TestName") -> ()  [unwired: 9 in, 1 out]
        n218 = property on="Progress" class="Clust (strict)"("Visible"=TRUE) -> ()  [unwired: 2 in, 2 out]
        n219 = property on="Motor" class="Clust (strict)"("Visible"=w336) -> ()  [unwired: 2 in, 2 out]
        n220 = property on="Test Slider" class="Slide (strict)"("Visible"=w336) -> ()  [unwired: 2 in, 2 out]
        n221 = property on="On/Off" class="Bool (strict)"("Visible"=w336) -> ()  [unwired: 2 in, 2 out]
        n222 = property on="Rev/Fwd" class="Clust (strict)"("Visible"=w336) -> ()  [unwired: 2 in, 2 out]
        n223 = property on="Test Ring" class="Ring (strict)"("Visible"=w336) -> ()  [unwired: 2 in, 2 out]
      }
      event "Command Selection": Value Change {
        # "Get the params and show in table"
        n224 = event-data() -> ("NewVal"=w346:i32)  [unwired: 1 in]
        n225 = property on="Command Selection" class="MCListbox (strict)"() -> ("ItemNames"=w344:string[][])  [unwired: 2 in, 2 out]
        n226 = call <vilib>:"WPI_DashboardUpdate Command Params.vi"("NewVal"=w346, "Commands"=w344, "Param Tbl"=w345) -> ()  [unwired: 8 in, 1 out]
      }
      event "Execute Command": Value Change {
        # "Started one, Unique ID holds\nresponse"
        n227 = event-data() -> ()  [unwired: 1 in, 1 out]
        n228 = property on="Command Selection" class="MCListbox (strict)"() -> ("ItemNames"=w357:string[][])  [unwired: 2 in, 2 out]
        n229 = Index Array(array=w357, index (row)="Command Selection", index (col)=0) -> (element=w355:string)
        n230 = call <vilib>:"Invoke Commands.vi"("Command Params"="Command Params", "Function Name"=w355) -> ("Params"=w351:u8, "Started"=w350:bool)  [unwired: 7 in, 1 out]
        n231 = Array Subset(array="Command Params", length (row)=w351) -> (w352:string[][])  [unwired: 3 in]
        n232 = Select(t="Executing" ("Cmd Status"), s=w350, f="" ("Cmd Status")) -> (s? t:f=→"Cmd Status":string)
      }
      event "Command Selection": Double Click {
        n233 = event-data() -> ("Row"=w365:i32)  [unwired: 1 in]
        n234 = property on="Command Selection" class="MCListbox (strict)"() -> ("ItemNames"=w368:string[][])  [unwired: 2 in, 2 out]
        n235 = local read "Command Params"() -> (w364:string[][])
        n236 = Index Array(array=w368, index (row)=w365, index (col)=0) -> (element=w366:string)
        n237 = call <vilib>:"Invoke Commands.vi"("Command Params"=w364, "Function Name"=w366) -> ("Params"=w363:u8, "Started"=w358:bool)  [unwired: 7 in, 1 out]
        n238 = Array Subset(array=w364, length (row)=w363) -> (w362:string[][])  [unwired: 3 in]
        n239 = Select(t="Executing" ("Cmd Status"), s=w358, f="" ("Cmd Status")) -> (s? t:f=w359:string)
        n240 = local write "Cmd Status"(w359) -> ()
      }
      event "CheckList": Double Click {
        # "Shift clears all"
        # "Update symbols on the listbox"
        n241 = event-data() -> ("PlatMods.Shift"=w370:bool, "Row"=w372:i32)  [unwired: 1 in]
        n242 = case shown="True" w370 {
          tunnel: w372 -> [w376 _]
          tunnel: 1 -> [w375 _]
          frame False {
            n243 = property on="CheckList" class="LstBox (strict)"() -> ("Item Symbols"=w374:i32[])  [unwired: 2 in, 2 out]
            n244 = Replace Array Subset(array=w374, new element=w375, index=w376) -> (w373:i32[])
            n245 = property on="CheckList" class="LstBox (strict)"("Item Symbols"=w373) -> ()  [unwired: 2 in, 2 out]
          }
          frame True {
            w377 = 0 ("Top Row")
            n246 = property on="CheckList" class="LstBox (strict)"() -> ("Number of Rows"=w379:u32)  [unwired: 2 in, 2 out]
            n247 = Initialize Array(0, w379) -> (w378:i32[])
            n248 = property on="CheckList" class="LstBox (strict)"("Top Row"=w377, "Value"=w377, "Item Symbols"=w378) -> ()  [unwired: 2 in, 2 out]
          }
        }
      }
      event "CheckList": Key Down {
        # "Update symbols on the listbox\nLeft and right keys check and uncheck"
        n249 = event-data() -> ("VKey"=w383:T28)  [unwired: 1 in]
        n250 = case shown="\"Left\", \"Right\"" w383 {
          selector: w383 -> [w388 _]
          tunnel: eventvkey."Left" ("VKey") -> [w386 _]
          frame "Left", "Right" {
            n251 = Equal?(x=w386, y=w388) -> (x = y?=w387:bool)
            n252 = Select(t=0, s=w387, f=1) -> (s? t:f=w389:i32)
            n253 = property on="CheckList" class="LstBox (strict)"() -> ("Item Symbols"=w392:i32[])  [unwired: 2 in, 2 out]
            n254 = Replace Array Subset(array=w392, new element=w389, index="CheckList") -> (w391:i32[])
            n255 = property on="CheckList" class="LstBox (strict)"("Item Symbols"=w391) -> ()  [unwired: 2 in, 2 out]
          }
          frame Default {
          }
        }
      }
      event "Motor.Enable": Value Change {
        # "When the test mode otor enable helper is set, update that\ntree row item's value"
        n256 = event-data() -> ("NewVal"=w398:bool)  [unwired: 1 in]
        n257 = Unbundle("Motor") -> ("Value"=w397:dbl)  [unwired: 1 out]
        n258 = Select(t=w397, s=w398, f=0.0) -> (s? t:f=w395:dbl)
        n259 = call <vilib>:"NT Write Number.vi"("Numeric"=w395, "Name"=w394) -> ()  [unwired: 9 in, 1 out]
      }
      event "Test Slider": Value Change {
        # "When the test mode slider helper is set, update that\ntree row item's value"
        n260 = event-data() -> ("NewVal"=w401:dbl)  [unwired: 1 in]
        n261 = call <vilib>:"NT Write Number.vi"("Numeric"=w401, "Name"=w402) -> ()  [unwired: 9 in, 1 out]
      }
      event "On/Off": Value Change {
        # "When the test mode on/off helper value is set, update that\ntree row item's value"
        n262 = event-data() -> ("NewVal"=w406:bool)  [unwired: 1 in]
        n263 = Boolean To (0,1)(Boolean=w406) -> (0, 1=w405:i16)
        n264 = call <vilib>:"NT Write Number.vi"("Numeric"=w405, "Name"=w404) -> ()  [unwired: 9 in, 1 out]
      }
      event "Rev/Fwd": Value Change {
        # "When the test mode helper value for relays is set, update that\ntree row item's value"
        n265 = event-data() -> ("NewVal.Forward"=w414:bool, "NewVal.Reverse"=w413:bool)  [unwired: 1 in]
        n266 = Boolean To (0,1)(Boolean=w414) -> (0, 1=w410:i16)
        n267 = Boolean To (0,1)(Boolean=w413) -> (0, 1=w412:i16)
        n268 = Negate(x=w412) -> (-x=w411:i16)
        n269 = Add(x=w410, y=w411) -> (x+y=w409:i16)
        n270 = call <vilib>:"NT Write Number.vi"("Numeric"=w409, "Name"=w408) -> ()  [unwired: 9 in, 1 out]
      }
      event "Test Ring": Value Change {
        # "When a test mode helper value is selected from the ring,\nset the tree item's variable to the string value"
        n271 = event-data() -> ("NewVal"=w418:u16)  [unwired: 1 in]
        n272 = property on="Test Ring" class="Ring (strict)"() -> ("Strings []"=w419:string[])  [unwired: 2 in, 2 out]
        n273 = Index Array(array=w419, index=w418) -> (element=w417:string)
        n274 = call <vilib>:"NT Write String.vi"("String"=w417, "Name"=w416) -> ()  [unwired: 9 in, 1 out]
      }
      event "Rec Mode": Value Change {
        # "Update globals for recording mode and path to read log from.\nClear when logging and let NetworkTables set path for vision to\nuse."
        n275 = event-data() -> ("NewVal"=w430:enum32{"Stop", "Record", "Playback"})  [unwired: 1 in]
        n276 = global write "WPI_DashboardLogging Global.vi" "Logging Filename"(path "") -> ()
        n277 = global write "WPI_DashboardLogging Global.vi" "Recording"(w430) -> ()
        n278 = case shown="\"Playback\"" w430 {
          tunnel: w429 -> [_ w432 w441]
          tunnel: [_ _ w440] -> w427
          tunnel: [_ _ w439] -> _
          tunnel: w425 -> [_ _ w437]
          tunnel: cluster{i32, i32} {-250, 170} -> [_ _ w436]
          tunnel: [_ _ T29 {"Image Size"=TRUE, "Image Type"=TRUE, "Pixel Value"=TRUE, "ROI Information"=TRUE, "Zoom Factor"=FALSE} ("Image Information Shown:All Elements")] -> w420
          tunnel: [_ _ TRUE ("Zoom Factor")] -> w421
          tunnel: w423 -> [_ _ w433]
          frame Default {
          }
          frame "Stop", "Record" {
            # "Place Window too"
            n279 = invoke class="VI" method="FP.Close"(reference=w432) -> (reference out=w431:refnum<vi>)  [unwired: 2 in, 2 out]
            n280 = invoke class="VI" method="Abort VI"(reference=w431) -> ()  [unwired: 2 in, 3 out]
          }
          frame "Playback" {
            n281 = call "Open Playback Panel.vi"("Offset"=w436, "DB VI Ref"=w437, "Playback in"=w441) -> ("Playback out"=w438:refnum<vi>)  [unwired: 8 in]
            n282 = register-events(w438, w433) -> (reference out=w440:refnum<event-registration>, error out=w439:errorcluster)  [unwired: 2 in]
          }
        }
        n283 = property on="Camera Image Right" class="ImageControl"("Image Information Shown"=w420, "Image Information Visible"=w421) -> ()  [unwired: 2 in, 2 out]
        n284 = property on="Camera Image" class="ImageControl"("Image Information Shown"=w420, "Image Information Visible"=w421) -> ()  [unwired: 2 in, 2 out]
        n285 = call <vilib>:"WPI_DashboardNT Log FieldName Cache.vi"("Operation"=enum16{"Lookup/Add", "Index", "Clear"}."Clear") -> ()  [unwired: 8 in, 3 out]
      }
      event Panel Close {
        w443 = enum32{"Stop", "Record", "Playback"}."Stop" ("Rec Mode")
        # "Playback window has been closed, abort"
        n286 = event-data() -> ()  [unwired: 1 in, 4 out]
        n287 = local write "Rec Mode"(w443) -> ()
        n288 = global write "WPI_DashboardLogging Global.vi" "Recording"(w443) -> ()
      }
      event Panel Close {
        # "Abort playback window and ourself"
        n289 = event-data() -> ()  [unwired: 1 in, 4 out]
        n290 = invoke class="VI" method="FP.Close"(reference=w447) -> (reference out=w446:refnum<vi>)  [unwired: 2 in, 2 out]
        n291 = invoke class="VI" method="Abort VI"(reference=w446) -> (error out=w445:errorcluster)  [unwired: 2 in, 2 out]
        n292 = invoke class="VI" method="Abort VI"(error in=w445) -> ()  [unwired: 2 in, 3 out]
      }
      event User Event {
        n293 = event-data() -> ("IDs"=w454:cluster{"RPC field ID":u16, "Unique ID":u16}, "String"=w453:string)  [unwired: 1 in]
        n294 = Bundle("IDs"=w454, "String"=w453) -> (w452:T13)  [unwired: 1 in]
        n295 = call <vilib>:"Retrieve RPC Response.vi"("RPC Response"=w452) -> ("Output"=w450:string[][])  [unwired: 10 in]
        n296 = Build Array (concatenate)(w448, w450) -> (w449:string[][])
        n297 = local write "Command Params"(w449) -> ()
        n298 = local write "Cmd Status"("" ("Cmd Status")) -> ()
      }
      event "Tree": Double Click {
        n299 = event-data() -> ("PlatMods"=w460:T32, "Tag"=w457:string)  [unwired: 1 in]
        n300 = Unbundle(w460) -> ("Shift"=w459:bool)  [unwired: 4 out]
        n301 = String Subset(string=w457, length (rest)=1 ("length (rest)")) -> (substring=w456:string)  [unwired: 1 in]
        n302 = Not(x=w459) -> (.not. x?=w458:bool)
        n303 = case shown="\"/\"" w456 {
          tunnel: w457 -> [_ w463]
          tunnel: w458 -> [_ w462]
          frame Default {
          }
          frame "/" {
            n304 = call <vilib>:"NT Update Persistence.vi"("Persistence"=w462, "Name"=w463) -> ()  [unwired: 9 in, 1 out]
          }
        }
      }
    }
  }
  n305 = while {
    tunnel: w61 -> [w465]
    i -> [w468]
    stop <- FALSE stop-if-true
    n306 = Wait (ms)(milliseconds to wait=u32 100) -> ()  [unwired: 1 out]
    n307 = case shown="\"Playback\"" "Rec Mode" {
      tunnel: w468 -> [_ _ w483]
      tunnel: [u32 2829099 ("Base Color") u32 11141120 ("Target Color") w472] -> w464
      frame "Stop", Default {
        # "Reset the color, extra updates don't cost much"
      }
      frame "Record" {
      }
      frame "Playback" {
        # "Playback"
        n308 = Quotient & Remainder(x=w483, y=u32 50 ("milliseconds to wait")) -> (x-y*floor(x/y)=w479:u32)  [unwired: 1 out]
        n309 = Divide(x=w479, y=u32 50 ("milliseconds to wait")) -> (x/y=w476:dbl)
        n310 = Multiply(x=6.283185307179586, y=w476) -> (x*y=w481:dbl)
        n311 = Sine(x=w481) -> (sin(x)=w480:dbl)
        n312 = Absolute Value(x=w480) -> (abs(x)=w473:dbl)
        n313 = call "Interpolate RGB Color.vi"("Proportion"=w473, "Target Color"=u32 30976, "Base Color"=u32 2829099) -> ("Result Color"=w472:u32)  [unwired: 8 in]
      }
    }
    n314 = property class="Pane"(reference=w465, "PaneColor"=w464) -> ()  [unwired: 1 in, 2 out]
  }
  n315 = local write "Dashboard Tab"(T2."Drive" ("Dashboard Tab")) -> ()
  n316 = property on="On/Off" class="Bool (strict)"("Visible"=w34) -> ()  [unwired: 2 in, 2 out]
  n317 = property on="Motor" class="Clust (strict)"("Visible"=w34) -> ()  [unwired: 2 in, 2 out]
  n318 = property on="Progress" class="Clust (strict)"("Visible"=w34) -> ()  [unwired: 2 in, 2 out]
  n319 = property on="Test Ring" class="Ring (strict)"("Visible"=w34) -> ()  [unwired: 2 in, 2 out]
  n320 = property on="Rev/Fwd" class="Clust (strict)"("Visible"=w34) -> ()  [unwired: 2 in, 2 out]
  n321 = while {
    tunnel: u16 1741 ("timeout ms (25000)") -> [w485]
    stop <- FALSE stop-if-true
    n322 = TCP Create Listener(10:w485) -> (0:w484:errorcluster, 3:w486:refnum<k5>)  [unwired: 4 in, 1 out]
    n323 = case shown="No Error" w484 {
      selector: w484 -> [w488 _]
      tunnel: w486 -> [w489 _]
      frame No Error {
        n324 = while {
          tunnel: w489 -> [w492]
          tunnel: w488 -> [w491]
          stop <- FALSE stop-if-true
          n325 = TCP Wait On Listener(8:w491, 11:w492) -> (0:w493:errorcluster, 4:w494:refnum<k5>)  [unwired: 2 in, 3 out]
          n326 = local write "TCP"(w494) -> ()
          n327 = case shown="No Error" w493 {
            frame No Error {
            }
            frame Error {
              n328 = Wait (ms)(milliseconds to wait=u32 1000) -> ()  [unwired: 1 out]
            }
          }
        }
      }
      frame Error {
        n329 = Wait (ms)(milliseconds to wait=u32 1000) -> ()  [unwired: 1 out]
      }
    }
  }
  n330 = while {
    stop <- FALSE stop-if-true
    n331 = disable-structure shown="Disabled" {
      frame Disabled {
        n332 = call-poly <vilib>:"NT Write Value.vi"("String"="Battery Number", "Name"="BatteryNumber") -> ()  [unwired: 9 in, 1 out]
      }
      frame Enabled {
      }
    }
    n333 = case shown="\"Do Front Right Cargo Ship\"" "Routine" {
      tunnel: [StartingLocation."Left Level 1" ("Starting Position") StartingLocation."Right Level 1" ("Starting Position") StartingLocation."Center Level 1" ("Starting Position") StartingLocation."Center Level 1" ("Starting Position") "Starting Position" StartingLocation."Center Level 1" ("Starting Position") StartingLocation."Center Level 1" ("Starting Position")] -> w517
      tunnel: [Piece."Hatch Panel" ("Starting Piece") Piece."Hatch Panel" ("Starting Piece") Piece."Hatch Panel" ("Starting Piece") Piece."Hatch Panel" ("Starting Piece") Piece."None" ("Starting Piece") Piece."Hatch Panel" ("Starting Piece") Piece."Hatch Panel" ("Starting Piece")] -> w513
      frame "Do Left Rocket", Default {
      }
      frame "Do Right Rocket" {
      }
      frame "Do Left Cargo Ship Panels" {
      }
      frame "Do Right Cargo Ship Panels" {
      }
      frame "Do Teleop" {
      }
      frame "Do Front Left Cargo Ship" {
      }
      frame "Do Front Right Cargo Ship" {
      }
    }
    "Starting Piece" <- w513
    n334 = call-poly <vilib>:"NT Read Value.vi"("Name"="ArmHeight") -> ("Numeric"=→"ArmHeight":dbl)  [unwired: 9 in, 1 out]
    n335 = call-poly <vilib>:"NT Read Value.vi"("Name"="LeftEncoder") -> ("Numeric"=→"LeftEncoder":dbl)  [unwired: 9 in, 1 out]
    n336 = call-poly <vilib>:"NT Write Value.vi"("Numeric"="Routine", "Name"="Routine") -> ()  [unwired: 9 in, 1 out]
    n337 = call-poly <vilib>:"NT Write Value.vi"("Numeric"="Rocket Level", "Name"="RocketLevel") -> ()  [unwired: 9 in, 1 out]
    n338 = call-poly <vilib>:"NT Write Value.vi"("Boolean"="Reset", "Name"="Reset") -> ()  [unwired: 9 in, 1 out]
    n339 = call-poly <vilib>:"NT Write Value.vi"("Numeric"="Delay", "Name"="Delay") -> ()  [unwired: 9 in, 1 out]
    n340 = call-poly <vilib>:"NT Read Value.vi"("Name"="LEDColorCode") -> ("Numeric"=w500:dbl)  [unwired: 9 in, 1 out]
    n341 = call-poly <vilib>:"NT Read Value.vi"("Name"="RightEncoder") -> ("Numeric"=→"RightEncoder":dbl)  [unwired: 9 in, 1 out]
    n342 = call-poly <vilib>:"NT Write Value.vi"("Numeric"="Pieces  to Score", "Name"="PiecesToScore") -> ()  [unwired: 9 in, 1 out]
    n343 = call-poly <vilib>:"NT Read Value.vi"("Name"="Gyro") -> ("Numeric"=→"Gyro":dbl)  [unwired: 9 in, 1 out]
    n344 = call-poly <vilib>:"NT Read Value.vi"("Name"="HatchLimitValue") -> ("Boolean"=→"HatchLimitSwitch":bool)  [unwired: 9 in, 1 out]
    n345 = call-poly <vilib>:"NT Read Value.vi"("Name"="LimitSwitchBottom") -> ("Boolean"=→"LimitSwitchBottom":bool)  [unwired: 9 in, 1 out]
    n346 = call-poly <vilib>:"NT Read Value.vi"("Name"="LimitSwitchTop") -> ("Boolean"=→"LimitSwitchTop":bool)  [unwired: 9 in, 1 out]
    n347 = call "LEDColorNumberToColor.vi"("ColorNumber"=w500) -> ("Color"=→"LEDs":u32)  [unwired: 10 in]
    n348 = Get Date/Time In Seconds() -> (seconds since 1Jan1904=w520:timestamp)
    n349 = Format Date/Time String(time format string (%c)="%Y-%m-%d_%H-%M", seconds (now)=w520) -> (date/time string=w521:string)  [unwired: 1 in]
    n350 = call-poly <vilib>:"NT Write Value.vi"("String"=w521, "Name"="DateandTime") -> ()  [unwired: 9 in, 1 out]
    n351 = local write "Starting Position"(w517) -> ()
    n352 = Wait (ms)(milliseconds to wait=u32 80) -> ()  [unwired: 1 out]
    n353 = call-poly <vilib>:"NT Write Value.vi"("Numeric"=w517, "Name"="StartingPosition") -> ()  [unwired: 9 in, 1 out]
  }
  n354 = local write "Command Selection"(u16 0 ("milliseconds to wait")) -> ()
  n355 = local write "Command Params"(string[][] [] ("Command Params")) -> ()
  n356 = global write "WPI_DashboardLogging Global.vi" "Recording"(w55) -> ()
  n357 = local write "Rec Mode"(w55) -> ()
  n358 = call <vilib>:"NT Write String.vi"("Name"="Auto Selector") -> ()  [unwired: 10 in, 1 out]
